vi "MTM2_registerCallback_command_startackcmd.vi"(8 "error in (no error)":errorcluster, 10 "skipOld":bool, 11 "handle":i32) -> (0 "error out":errorcluster, 3 "function return":i32)   [LabVIEW 2018, in "SALLV_MTM2.lvlib"]
doc: "int MTM2_shm_registerCallback_command_start_ackcmdLV(int handle, bool skipOld);"
uses:
  SALLV_MTM2.lvlib
  SALLV_MTM2.so
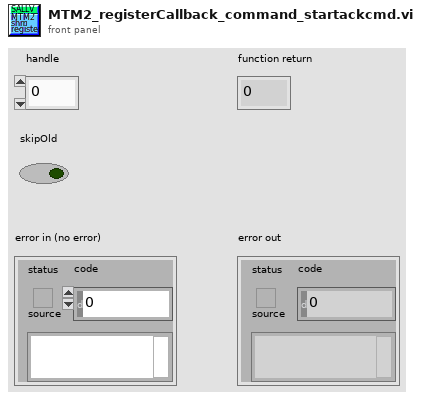
[diagram p1: front panel]
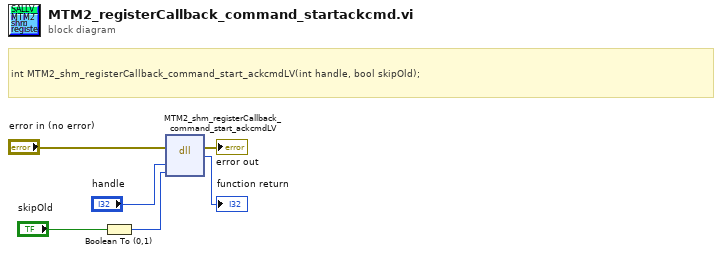
[diagram p0: block diagram]
diagram:
  # "int MTM2_shm_registerCallback_command_start_ackcmdLV(int handle, bool skipOld);"
  n1 = Boolean To (0,1)(Boolean="skipOld") -> (0, 1=w3:i16)
  n2 = dll-call lib="home/ttsai/Document/salApiMTM2/SALLV_MTM2/SALLV_MTM2.*" fn="MTM2_shm_registerCallback_command_start_ackcmdLV"(error in="error in (no error)", "handle"="handle", "skipOld"=w3) -> (error out=→"error out":errorcluster, →"function return":i32)  [unwired: 4 in, 1 out]
